vi "Sending_Seek_Recipe_With_Seek_Cmd_SUB_VI.vi"(0 "connection ID - In":refnum<k5>, 3 "Receipe Msg ID":i32=65, 4 "Receipe Message length":i32=36, 5 "Response ID":u8=66, 6 "MemoryClearBeforeSeek":i32, 7 "error in (no error)":errorcluster, 8 "SeekTime":i32=500, 9 "SeekFreqLimitLow":i32=500, 10 "SeekAmplitudeLoopC2":i32=300, 12 "SeekAmplitudeLoopC1":i32=100, 13 "SeekPhaseloopI":i32=450, 15 "SeekPhaseloopCF":i32=450, 16 "SeekFreqLimitHigh":i32=500, 17 "SeekRampTime":i32=500, 20 "SeekFreqOffset":i32) -> (18 "connection ID out":refnum<k5>, 22 "End Frequency and Time Stamp":string, 25 "SEEK recipe Parameter range validation":string, 27 "error out":errorcluster)   [LabVIEW 2017]
panel:
  out "bytes written":i32
  # "OUTPUT"
  # "INPUT"
  # "Parameter Name                      20KHz                                                                                                          \t40KHz\t\t\n\t                                    Default Value\t    Min Value\t       Max Value\t                                     Default Value         \tMin Value\t            Max Value\nSeek Time                            \t500                  \t1                     \t500\t                                                                500\t        1\t                               500\nAmplitude loop C1\t             100\t                   1                    \t20000\t                                                           \t100\t          1                             20000\nAmplidute Loop C2\t             300                   \t1\t                    20000\t                                                           \t300\t           1                          \t20000\nFreq Limit High\t                     500\t                 1\t                      100\t                                                                 \t500\t         1                          \t100\nFreq Limit Low\t                        500\t                1\t                      100\t                                                                500\t         1                            \t100\nPhase Loop\t                           450\t                 50                       500\t                                                            \t450\t           50\t                           500\nPhaser Loop CF                   \t450                  \t50\t                       500\t                                                              \t450        \t50\t                            500\nRamp Time                          \t500\t                  300\t                    700\t                                                                 \t500          300\t                        700\nFreq Offset\t                               0\t                  0\t                        20\t                                                                        \t0\t         0\t                            20\nMemoryClearBeforeSeek        0                   0                         1                                                                         0             0                              1"
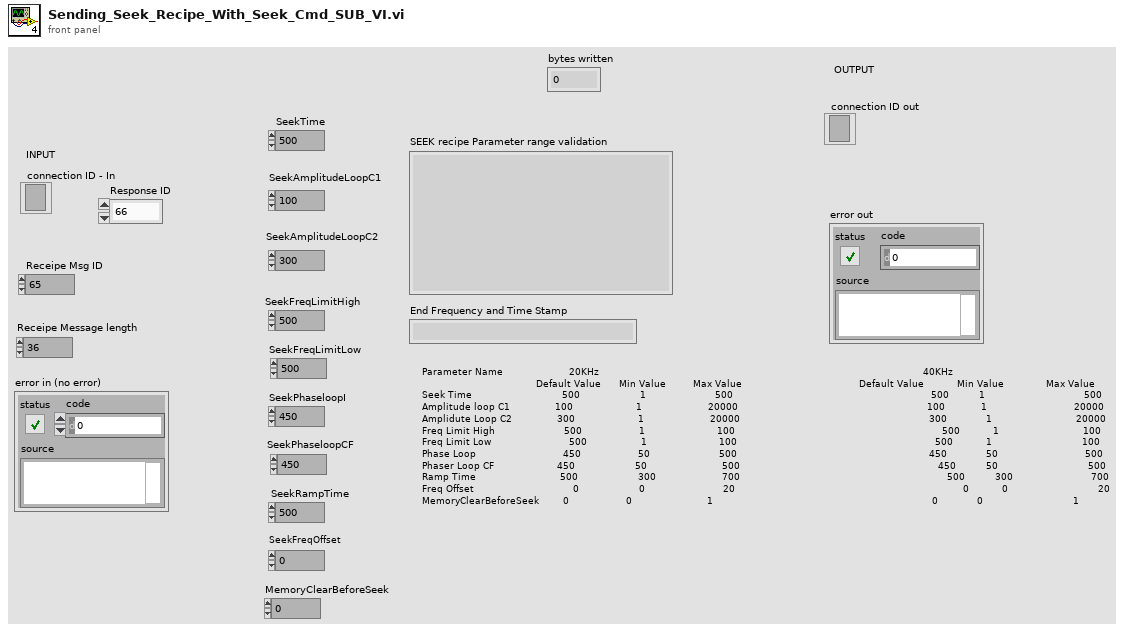
[diagram p1: front panel]
types:
  T1 = enum16{"Standard", "Buffered", "CRLF", "Immediate"}
  T2 = cluster{"Seek Request Message Length to DB ":i64, "Seek Request Message ID to DB":i64}
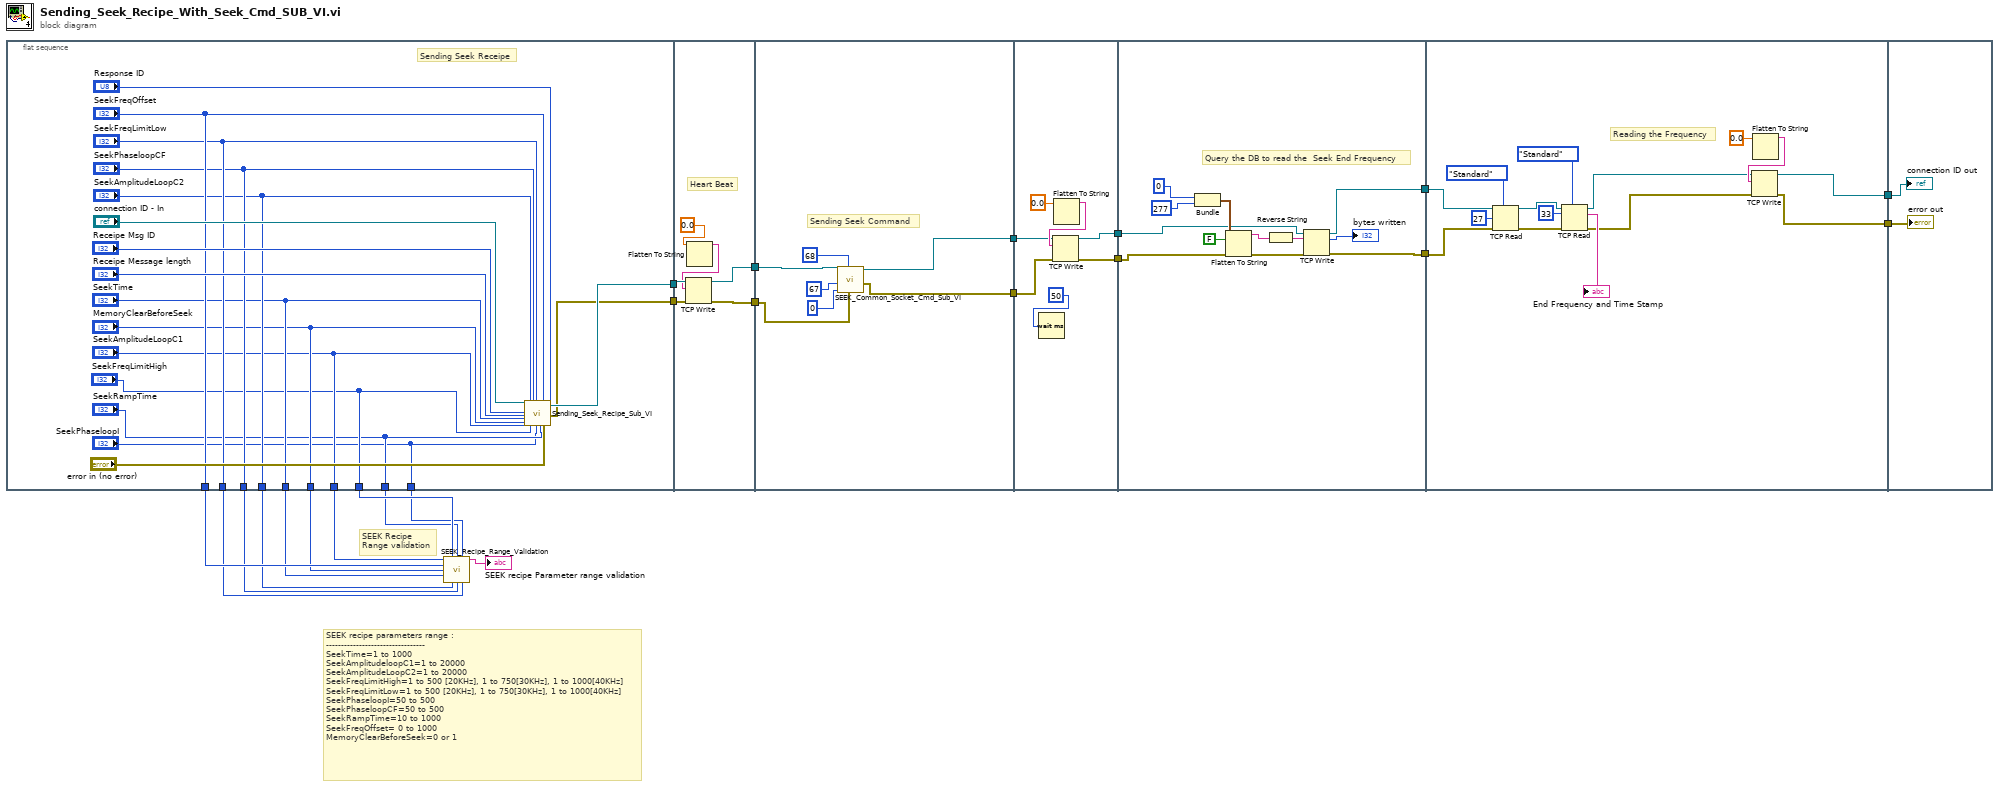
[diagram p0: block diagram]
diagram:
  # "SEEK Recipe \nRange validation"
  # "SEEK recipe parameters range :\n--------------------------------- \nSeekTime=1 to 1000\nSeekAmplitudeloopC1=1 to 20000\nSeekAmplitudeLoopC2=1 to 20000\nSeekFreqLimitHigh=1 to 500 [20KHz], 1 to 750[30KHz], 1 to 1000[40KHz]\nSeekFreqLimitLow=1 to 500 [20KHz], 1 to 750[30KHz], 1 to 1000[40KHz]\nSeekPhaseloopI=50 to 500\nSeekPhaseloopCF=50 to 500\nSeekRampTime=10 to 1000\nSeekFreqOffset= 0 to 1000\nMemoryClearBeforeSeek=0 or 1"
  n1 = flat-sequence {
    tunnel: [w40] -> w23
    tunnel: [w39] -> w22
    tunnel: ["SeekFreqOffset"] -> w13
    tunnel: ["SeekFreqLimitLow"] -> w12
    tunnel: ["SeekPhaseloopCF"] -> w11
    tunnel: ["SeekAmplitudeLoopC2"] -> w10
    tunnel: ["SeekTime"] -> w9
    tunnel: ["MemoryClearBeforeSeek"] -> w8
    tunnel: ["SeekAmplitudeLoopC1"] -> w7
    tunnel: ["SeekFreqLimitHigh"] -> w6
    tunnel: ["SeekRampTime"] -> w5
    tunnel: ["SeekPhaseloopI"] -> w4
    tunnel: w23 -> [w46]
    tunnel: w22 -> [w45]
    tunnel: [w43] -> w21
    tunnel: [w44] -> w20
    tunnel: w21 -> [w53]
    tunnel: w20 -> [w52]
    tunnel: [w51] -> w18
    tunnel: [w50] -> w16
    tunnel: w18 -> [w56]
    tunnel: [w55] -> w17
    tunnel: w16 -> [w57]
    tunnel: [w54] -> w15
    tunnel: w17 -> [w66]
    tunnel: w15 -> [w67]
    tunnel: [w68] -> w2
    tunnel: [w65] -> w1
    tunnel: w2 -> [w76]
    tunnel: w1 -> [w75]
    tunnel: [w82] -> w19
    tunnel: [w83] -> w14
    tunnel: w19 -> [w89]
    tunnel: w14 -> [w88]
    frame #0 {
      # "Sending Seek Receipe"
      n2 = call "Sending_Seek_Recipe_Sub_VI.vi"("connection ID"="connection ID - In", "Receipe Msg ID"="Receipe Msg ID", "Receipe Message length"="Receipe Message length", "SeekTime"="SeekTime", "MemoryClearBeforeSeek"="MemoryClearBeforeSeek", "SeekAmplitudeLoopC1"="SeekAmplitudeLoopC1", "SeekAmplitudeLoopC2"="SeekAmplitudeLoopC2", "SeekFreqLimitHigh"="SeekFreqLimitHigh", "SeekPhaseloopCF"="SeekPhaseloopCF", "SeekFreqLimitLow"="SeekFreqLimitLow", "SeekPhaseloopI"="SeekPhaseloopI", "SeekRampTime"="SeekRampTime", "SeekFreqOffset"="SeekFreqOffset", "error input"="error in (no error)", "Response ID"="Response ID") -> ("connection ID"=w40:refnum<k5>, "error out"=w39:errorcluster)  [unwired: 11 in]
    }
    frame #1 {
      # "Heart Beat"
      n3 = Flatten To String(anything=0.0) -> (data string=w41:string)  [unwired: 3 in, 2 out]
      n4 = TCP Write(connection ID=w46, data in=w41, error in (no error)=w45) -> (connection ID out=w43:refnum<k5>, error out=w44:errorcluster)  [unwired: 1 in, 1 out]
    }
    frame #2 {
      # "Sending Seek Command"
      n5 = call "SEEK_Common_Socket_Cmd_Sub_VI.vi"("Common Socket Error in"=w52, "Response ID 1"=u8 68, "Operation Message Length 1"=0, "Operation Message ID 1"=67, "connection ID"=w53) -> ("error out"=w51:errorcluster, "connection ID"=w50:refnum<k5>)  [unwired: 4 in, 1 out]
    }
    frame #3 {
      n6 = Wait (ms)(milliseconds to wait=u32 50) -> ()  [unwired: 1 out]
      n7 = Flatten To String(anything=0.0) -> (data string=w58:string)  [unwired: 3 in, 2 out]
      n8 = TCP Write(connection ID=w57, data in=w58, error in (no error)=w56) -> (connection ID out=w54:refnum<k5>, error out=w55:errorcluster)  [unwired: 1 in, 1 out]
    }
    frame #4 {
      # "Query the DB to read the  Seek End Frequency"
      n9 = Bundle("Seek Request Message Length to DB"=i64 0, "Seek Request Message ID to DB"=i64 277) -> (w69:T2)  [unwired: 1 in]
      n10 = Flatten To String(anything=w69, prepend array or string size? (T)=FALSE, error in (no error)=w66) -> (data string=w72:string, error out=w71:errorcluster)  [unwired: 1 in, 1 out]
      n11 = Reverse String(1:w72) -> (0:w63:string)
      n12 = TCP Write(connection ID=w67, data in=w63, error in (no error)=w71) -> (connection ID out=w68:refnum<k5>, bytes written=→"bytes written":i32, error out=w65:errorcluster)  [unwired: 1 in]
    }
    frame #5 {
      # "Reading the Frequency"
      n13 = TCP Read(connection ID=w76, bytes to read=27, error in (no error)=w75, 7:T1."Standard" ("mode (standard)")) -> (connection ID out=w78:refnum<k5>, error out=w77:errorcluster)  [unwired: 1 in, 1 out]
      n14 = TCP Read(connection ID=w78, bytes to read=33, error in (no error)=w77, 7:T1."Standard" ("mode (standard)")) -> (connection ID out=w80:refnum<k5>, data out=→"End Frequency and Time Stamp":string, error out=w79:errorcluster)  [unwired: 1 in]
      n15 = Flatten To String(anything=0.0) -> (data string=w84:string)  [unwired: 3 in, 2 out]
      n16 = TCP Write(connection ID=w80, data in=w84, error in (no error)=w79) -> (connection ID out=w82:refnum<k5>, error out=w83:errorcluster)  [unwired: 1 in, 1 out]
    }
    frame #6 {
      "error out" <- w88
      "connection ID out" <- w89
    }
  }
  n17 = call "SEEK_Recipe_Range_Validation.vi"("SeekAmplitudeLoopC1"=w7, "SeekFreqLimitHigh"=w6, "SeekRampTime"=w5, "SeekPhaseloopI"=w4, "SeekFreqOffset"=w13, "MemoryClearBeforeSeek"=w8, "SeekTime"=w9, "SeekAmplitudeLoopC2"=w10, "SeekPhaseloopCF"=w11, "SeekFreqLimitLow"=w12) -> ("String"=→"SEEK recipe Parameter range validation":string)  [unwired: 5 in]
